vi "BUILD_install dependencies.vi"() -> ()   [LabVIEW 2013]
panel:
  out "error out":errorcluster
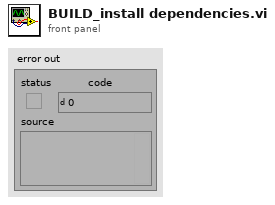
[diagram p1: front panel]
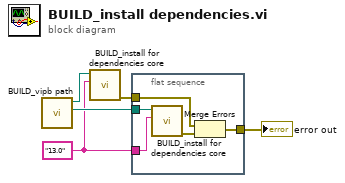
[diagram p0: block diagram]
diagram:
  w1 = "13.0" ("LabVIEW Version")
  n1 = call "BUILD_vipb path.vi"() -> ("2"=w2:path, "appended path"=w5:path)  [unwired: 10 in]
  n2 = call "BUILD_install for dependencies core.vi"("LabVIEW Version"=w1, "vipb path"=w5) -> ("error out"=w4:errorcluster)  [unwired: 9 in]
  n3 = flat-sequence {
    tunnel: w4 -> [w10]
    tunnel: [w9] -> w3
    tunnel: w2 -> [w7]
    tunnel: w1 -> [w6]
    frame #0 {
      n4 = call "BUILD_install for dependencies core.vi"("LabVIEW Version"=w6, "vipb path"=w7) -> ("error out"=w8:errorcluster)  [unwired: 9 in]
      n5 = Merge Errors(w10, w8) -> (w9:errorcluster)
    }
  }
  "error out" <- w3
